vi "Connection - COPT Connection Request.vi"(8 "error in (no error)":errorcluster, 11 "S7NetCom in":refnum<class "S7NetCom.lvclass">) -> (0 "error out":errorcluster, 2 "TPDU":u8[](array[numeric]), 3 "S7NetCom out":refnum<class "S7NetCom.lvclass">)   [LabVIEW 2014, in "S7NetCom.lvclass"]
doc: "____\nCopyright (c) 2019 Hampel Software Engineering (HSE), released under BSD license. More info can be found on https://dokuwiki.hampel-soft.com/code/hse/s7netcom. Original code published by Marc Christenson, Sisu Devices."
uses:
  S7NetCom.lvclass
  S7NetCom.lvclass/S7NetCom.ctl
  TPKT/TPKT - Add Header.vi
  Accessors/Get Timeout.vi
  Accessors/Get TCP Ref.vi
  Accessors/Set TCP Ref.vi
  TPKT/TPKT - Header Bytes 1 and 2--constant.vi
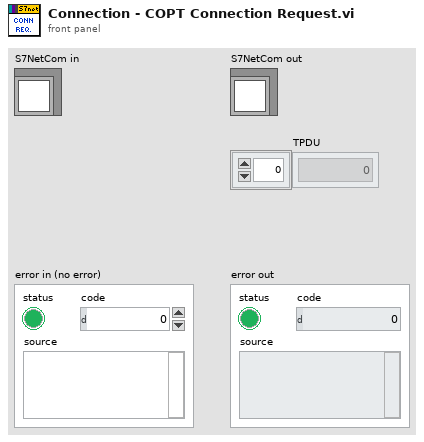
[diagram p1: front panel]
types:
  T1 = typedef "S7NetCom.lvclass/S7NetCom_HexByteArray.ctl" = T2[]
  T2 = typedef "S7NetCom.lvclass/S7NetCom_HexByte.ctl" = u8
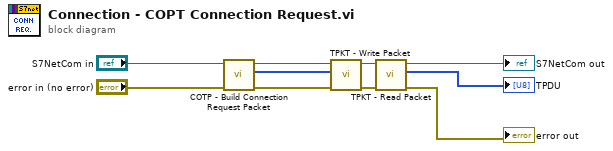
[diagram p0: block diagram]
diagram:
  n1 = call "COTP - Build Connection Request Packet.vi"("error in (no error)"="error in (no error)", "S7NetCom in"="S7NetCom in") -> ("error out"=w10:errorcluster, "COTP Connection Request"=w1:T1, "S7NetCom out"=w8:refnum<class "S7NetCom.lvclass">)  [unwired: 7 in]
  n2 = call "TPKT - Write Packet.vi"("error in"=w10, "TPDU"=w1, "S7"=w8) -> ("error out"=w2:errorcluster, "S7 out"=w4:refnum<class "S7NetCom.lvclass">)  [unwired: 7 in]
  n3 = call "TPKT - Read Packet.vi"("error in (no error)"=w2, "S7"=w4) -> ("error out"=→"error out":errorcluster, "TPDU"=→"TPDU":T1, "S7 out"=→"S7NetCom out":refnum<class "S7NetCom.lvclass">)  [unwired: 7 in]
